vi "AMWave.vi"() -> ()   [LabVIEW 2014]
uses:
  <vilib>/imath/engines/lvmath2/RunTimeEngine/Managers/WorkSpace/UID Generator.vi
  <vilib>/imath/engines/lvmath2/RunTimeEngine/RunTimeType/NIMS_RunTimeType_From StrictType (excl LVString).vi
  <instcachedir>/0/NIMS_RunTimeType_From StrictType (excl LVString)_15A5391EEA9C4AACB9955AC755B83D29.lvgen/NIMS_RunTimeType_From StrictType (excl LVString)_15A5391EEA9C4AACB9955AC755B83D29_000.vi
  <vilib>/imath/engines/lvmath2/RunTimeEngine/LocalVariableDefStatement/MC_LocalVariableDefStatement_Display.vi
  <vilib>/imath/engines/lvmath2/RunTimeEngine/RangeToken/NIMS_Range.vi
  <instcachedir>/0/NIMS_Range_9BCE657718DF4976A877346C61F22738.lvgen/NIMS_Range_9BCE657718DF4976A877346C61F22738_000.vi
  <vilib>/imathl/engines/lvmath/Functions/Error Handling/Create Error.vi
  <vilib>/imath/engines/lvmath2/RunTimeEngine/ArithmeticOperatorToken/NIMS_ArithmeticOperator_times.vi
  <instcachedir>/0/NIMS_ArithmeticOperator_times_2EFF5B13FCA4492A81D59089AD809F54.lvgen/NIMS_ArithmeticOperator_times_2EFF5B13FCA4492A81D59089AD809F54_000.vi
  <vilib>/imath/engines/lvmath2/RunTimeEngine/Managers/SymbolTable/Clear UID.vi
  <vilib>/imath/engines/lvmath2/RunTimeEngine/NodeEndStatement/NIMS_NodeEndStatement_Output.vi
  <instcachedir>/0/NIMS_NodeEndStatement_Output_53EC0D466D134D7ABD903AC30B43404B.lvgen/NIMS_NodeEndStatement_Output_53EC0D466D134D7ABD903AC30B43404B_005.vi
  <vilib>/imath/engines/lvmath2/RunTimeEngine/ErrorHandling/NIMS_Finalize Error.vi
  <vilib>/imath/engines/lvmath2/RunTimeEngine/Managers/SymbolTable/NIMS_WorkSpace.lvlib
panel:
  out "XY Graph 2":cluster{"t":dbl[], "x":dbl[]}(graph)
  out "AM waves":cluster{"Time":dbl[], "Displacement":dbl[]}
  in  "AM Wave parameters":T1
  in  "Digitalizing Parameters":T2
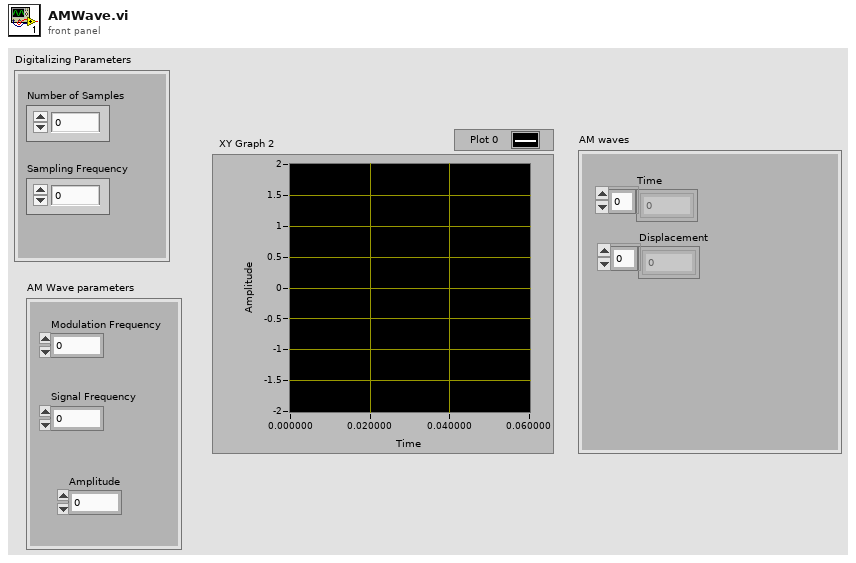
[diagram p1: front panel]
types:
  T1 = cluster{"Signal Frequency":dbl, "Amplitude":dbl, "Modulation Frequency":dbl}
  T2 = cluster{"Number of Samples":dbl, "Sampling Frequency":dbl}
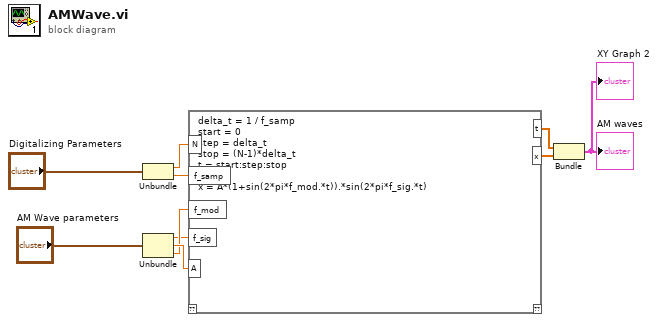
[diagram p0: block diagram]
diagram:
  n1 = Unbundle("Digitalizing Parameters") -> ("Number of Samples"=w9:dbl, "Sampling Frequency"=w8:dbl)
  n2 = Unbundle("AM Wave parameters") -> ("Signal Frequency"=w4:dbl, "Amplitude"=w6:dbl, "Modulation Frequency"=w5:dbl)
  n3 = mathscript code="delta_t = 1 / f_samp\nstart = 0\nstep = delta_t\nstop = (N-1)*delta_t\nt = start:step:stop\n\nx = A*(1+sin(2*pi*f_mod.*t)).*sin(2*pi*f_sig.*t)"("N"=w9, "f_samp"=w8, "f_mod"=w5, "f_sig"=w4, "A"=w6) -> ("x"=w2:dbl[], "t"=w3:dbl[])  [unwired: 1 in, 1 out]
  n4 = Bundle("t"=w3, "x"=w2) -> (→"AM waves" →"XY Graph 2":cluster{"t":dbl[], "x":dbl[]})  [unwired: 1 in]
